vi "GEA2 Send and Receive Message.vi"(0 "GEA2 Reference In":refnum<k24>, 1 "Input Data":T1 {"Command" format="%02x"; "Destination" format="%02x"; "Source" format="%02x"}, 2 "Read Timeout (ms)":u32=500, 5 "Expected Command":string=".*", 7 "Expected Data":string=".*", 9 "Expected Data 2":string, 11 "Error In":errorcluster, 13 "Expected Command 2":string=".*", 14 "Disable Expected Data":bool) -> (4 "GEA2 Reference Out":refnum<k24>, 6 "Raw Data Out":string, 8 "Converted Data Out":T2 {"CRC" format="%04x"; "Length" format="%02x"; "Command" format="%02x"; "Destination" format="%02x"; "Source" format="%02x"}, 15 "Error Out":errorcluster)   [LabVIEW 2014, in "GEA2_Toolkit.lvlib"]
doc: "This VI sends and receives data across the GEA2 bus. The VI waits for the expected responses (filtered by the expected command / data fields) or until the timeout occurs."
uses:
  library/GEA2_Toolkit.lvlib
  C:/Automation/DLLs/PC Tools .NET/GeaCommunication.dll
  Automation/DLLs/PC Tools .NET/GeaCommunication.dll
  type defs/Data In.ctl
  type defs/Data Out.ctl
panel:
  out "error IO":errorcluster
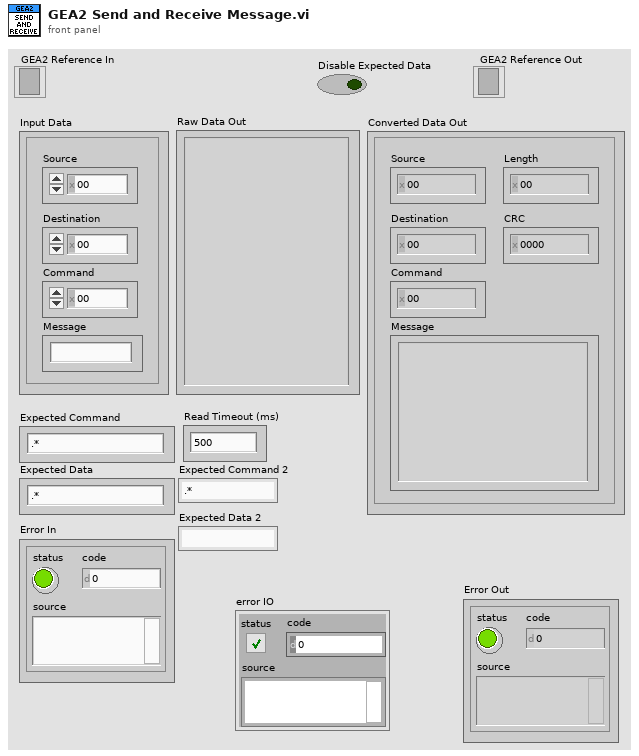
[diagram p1: front panel]
types:
  T1 = typedef "GEA2_Toolkit.lvlib/Data In.ctl" = cluster{"Source":u8, "Destination":u8, "Command":u8, "Message":string}
  T2 = typedef "GEA2_Toolkit.lvlib/Data Out.ctl" = cluster{"Source":u8, "Destination":u8, "Command":u8, "Length":u8, "CRC":u16, "Message":string}
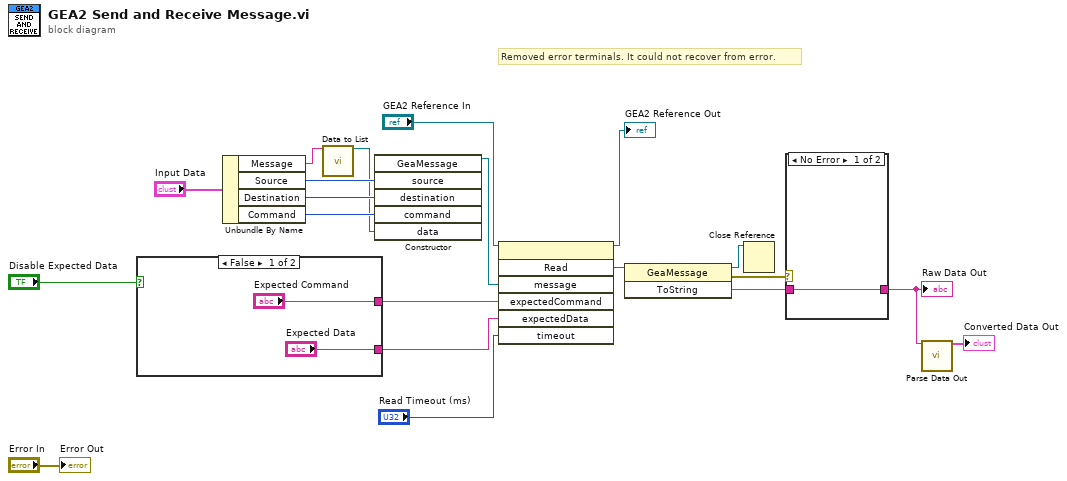
[diagram p0: block diagram]
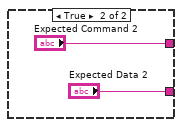
[diagram p2: hidden frame]
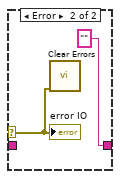
[diagram p3: hidden frame]
diagram:
  # "Removed error terminals. It could not recover from error."
  n1 = case shown="False" "Disable Expected Data" {
    tunnel: ["Expected Data" "Expected Data 2"] -> w17
    tunnel: ["Expected Command" "Expected Command 2"] -> w16
    frame False {
    }
    frame True {
    }
  }
  n2 = Unbundle By Name("Input Data") -> ("Message"=w11:string, "Source"=w10:u8, "Destination"=w9:u8, "Command"=w8:u8)
  n3 = call "Data to List.vi"("Data String In"=w11) -> ("Data List Out"=w7:refnum<k24>)  [unwired: 13 in, 1 out]
  n4 = constructor class="GeaMessage"("source"=w10, "destination"=w9, "command"=w8, "data"=w7) -> (reference out=w1:refnum<k24>)  [unwired: 3 in, 6 out]
  n5 = invoke method="Read"(reference="GEA2 Reference In", "message"=w1, "expectedCommand"=w16, "expectedData"=w17, "timeout"="Read Timeout (ms)") -> (reference out=→"GEA2 Reference Out":refnum<k24>, "Read"=w6:refnum<k24>)  [unwired: 2 in, 5 out]
  n6 = invoke class="GeaMessage" method="ToString"(reference=w6) -> (reference out=w14:refnum<k24>, error out=w13:errorcluster, "ToString"=w12:string)  [unwired: 2 in]
  n7 = Close Reference(reference=w14) -> ()  [unwired: 1 in, 1 out]
  n8 = case shown="No Error" w13 {
    selector: w13 -> [_ w26]
    tunnel: w12 -> [w25 _]
    tunnel: [w25 "" ("ToString")] -> w19
    frame No Error {
    }
    frame Error {
      n9 = call <vilib>:"Clear Errors.vi"("error in (no error)"=w26) -> ()  [unwired: 5 in, 2 out]
      "error IO" <- w26
    }
  }
  "Raw Data Out" <- w19
  n10 = call "Parse Data Out.vi"("Raw Data In"=w19) -> ("Data Out"=→"Converted Data Out":T2)  [unwired: 13 in, 1 out]
  "Error Out" <- "Error In"
